vi "Start Sync.vi"(8 "error in (no error)":errorcluster, 11 "gRPC Server in":refnum<class "Greeter.lvclass">) -> (0 "error out":errorcluster, 3 "gRPC Server out":refnum<class "Greeter.lvclass">)   [LabVIEW 2019, in "helloworld_server.lvlib" / "Greeter.lvclass"]
uses:
  Greeter.lvclass
  Greeter.lvclass/Greeter.ctl
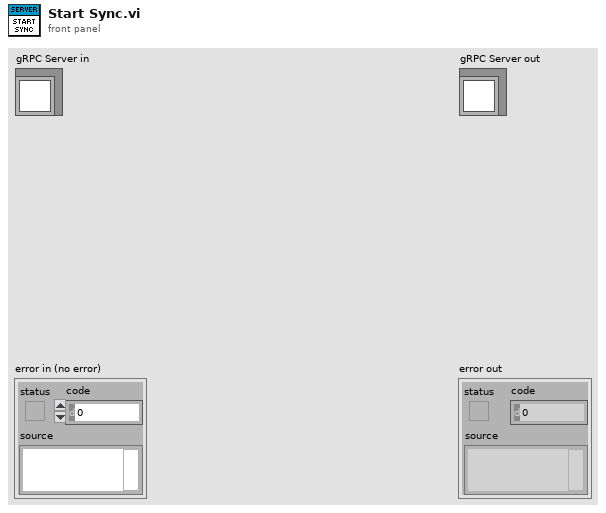
[diagram p1: front panel]
types:
  T1 = typedef "helloworld_server.lvlib/Greeter.lvclass/Server Internal UEs.ctl" = cluster{"helloworld_Greeter_SayHello Internal UE":refnum<user-event>}
  T2 = typedef "helloworld_server.lvlib/Greeter.lvclass/Server gRPC UEs.ctl" = cluster{"helloworld_Greeter_SayHello gRPC UE":refnum<user-event>}
  T3 = typedef "gprc-lvsupport-release.lvlib/grpcId.ctl" = u64
  T4 = typedef "helloworld_server.lvlib/helloworld_HelloRequest.ctl" = cluster{"name":string}
  T5 = typedef "grpc-lvsupport-release.lvlib/grpcId.ctl" = u64
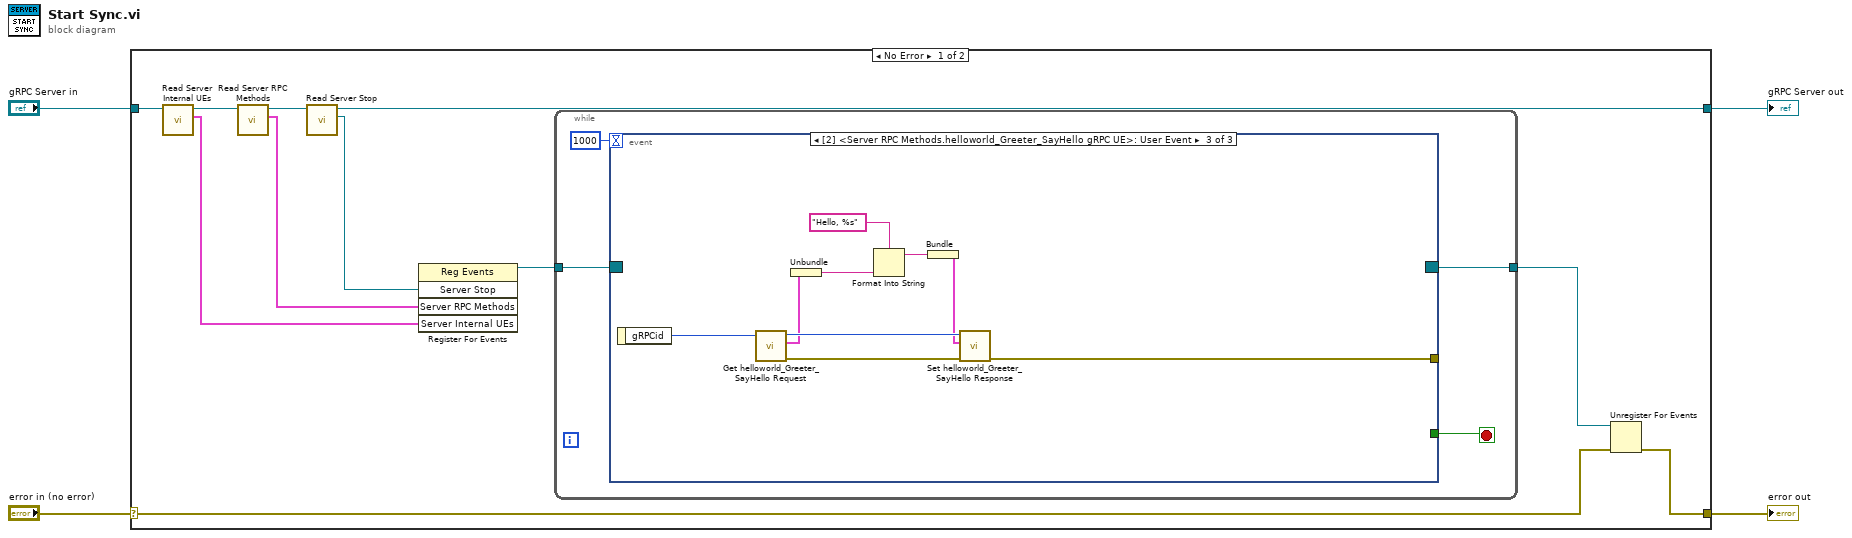
[diagram p0: block diagram]
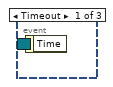
[diagram p2: hidden frame]
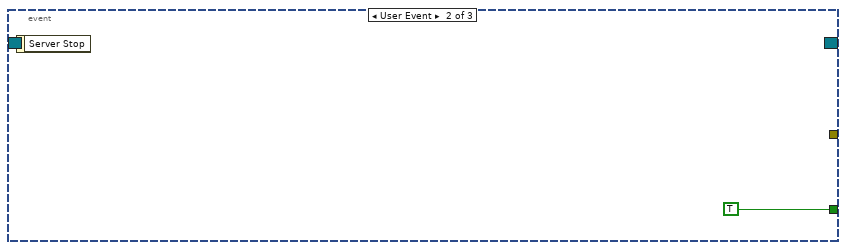
[diagram p3: hidden frame]
diagram:
  n1 = case shown="No Error" "error in (no error)" {
    selector: "error in (no error)" -> [w9 w31]
    tunnel: [w8 w31] -> w3
    tunnel: [w6 w30] -> w1
    tunnel: "gRPC Server in" -> [w15 w30]
    frame No Error {
      n2 = call "Read Server Internal UEs.vi"("SignalGeneratorService in"=w15) -> ("Server Internal UEs"=w13:T1, "SignalGeneratorService out"=w14:refnum<class "Greeter.lvclass">)  [unwired: 8 in, 1 out]
      n3 = call "Read Server RPC Methods.vi"("SignalGeneratorService in"=w14) -> ("Server RPC Methods"=w7:T2, "SignalGeneratorService out"=w12:refnum<class "Greeter.lvclass">)  [unwired: 8 in, 1 out]
      n4 = call-dynamic "Read Server Stop.vi"("iService in"=w12) -> ("Server Stop"=w5:refnum<user-event>, "iService out"=w6:refnum<class "Greeter.lvclass">)  [unwired: 8 in, 1 out]
      n5 = register-events(w5, w7, w13) -> (reference out=w11:refnum<event-registration>)  [unwired: 2 in, 1 out]
      n6 = while {
        tunnel: w11 -> [w19]
        tunnel: [w17] -> w10
        stop <- w18 stop-if-true
        n7 = event "RPC Methods Event Structure" shown="[2] <Server RPC Methods.helloworld_Greeter_SayHello gRPC UE>: User Event" {
          selector: w19 -> [_ _ _]
          dyn-events: [_ _ _] -> w17
          timeout: 1000 -> [_ _ _]
          tunnel: [_ TRUE _] -> w18
          tunnel: [_ _ w26] -> _
          event Timeout {
            n8 = event-data() -> ()  [unwired: 1 in, 1 out]
          }
          event User Event {
            n9 = event-data() -> ()  [unwired: 1 in, 1 out]
          }
          event User Event {
            n10 = event-data() -> ("gRPCid"=w29:T3)  [unwired: 1 in]
            n11 = call "Get helloworld_Greeter_SayHello Request.vi"("gRPCid in"=w29) -> ("error out"=w27:errorcluster, "Message Data"=w25:T4, "gRPCid out"=w28:T5)  [unwired: 8 in]
            n12 = Unbundle(w25) -> ("name"=w23:string)
            n13 = Format Into String(format string="Hello, %s", w23) -> (resulting string=w21:string)  [unwired: 2 in, 1 out]
            n14 = Bundle(w21) -> (w24:cluster{string})  [unwired: 1 in]
            n15 = call "Set helloworld_Greeter_SayHello Response.vi"("error in (no error)"=w27, "Message Data"=w24, "gRPCid in"=w28) -> ("error out"=w26:errorcluster)  [unwired: 8 in]
          }
        }
      }
      n16 = Unregister For Events(event registration refnum=w10, error in=w9) -> (error out=w8:errorcluster)
    }
    frame Error {
    }
  }
  "error out" <- w3
  "gRPC Server out" <- w1
